vi "SaveBackground.vi"(8 "error in (no error)":errorcluster, 10 "Path":path, 11 "Background In":T1=refnum) -> (0 "error out":errorcluster, 3 "Background Out":T1)   [LabVIEW 2019]
uses:
  <vilib>/vision/Image Controls.llb/IMAQ Image.ctl
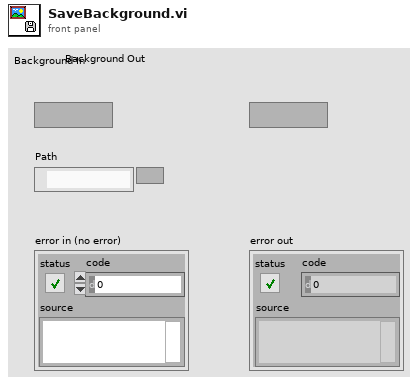
[diagram p1: front panel]
types:
  T1 = typedef "IMAQ Image.ctl" = refnum<image>
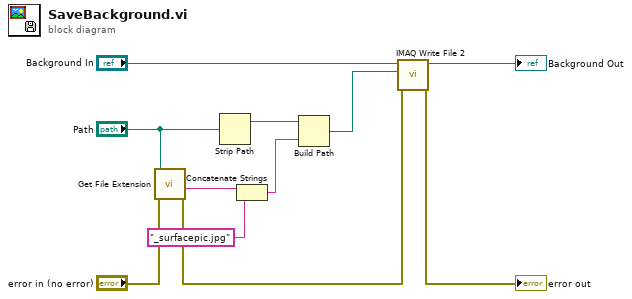
[diagram p0: block diagram]
diagram:
  n1 = call <vilib>:"Get File Extension.vi"("error in (no error)"="error in (no error)", "file"="Path") -> ("error out"=w5:errorcluster, "filename without extension"=w3:string)  [unwired: 5 in, 3 out]
  n2 = Strip Path(path="Path") -> (stripped path=w11:path)  [unwired: 1 out]
  n3 = Concatenate Strings(w3, "_surfacepic.jpg" ("string")) -> (w1:string)
  n4 = Build Path(base path=w11, name or relative path=w1) -> (appended path=w10:path)
  n5 = call-poly "IMAQ Write File 2"("error in (no error)"=w5, "File Path"=w10, "Image"="Background In") -> ("error out"=→"error out":errorcluster, "Image Out (duplicate)"=→"Background Out":T1)  [unwired: 7 in]
